vi "build_PWM_task.vi"(0 "counter":string="Dev1/ctr0", 1 "idle state":i32(ring)=10214 items=["High"=10192, "Low"=10214], 2 "initial delay":dbl format="%^.2e", 3 "sample mode":i32(ring)=10178 items=["Finite Samples"=10178, "Continuous Samples"=10123, "Hardware Timed Single Point"=12522], 5 "channel name":string="pwm out", 7 "low time":dbl=0.01 format="%0.2e", 9 "high time":dbl=0.01 format="%0.2e", 11 "error in":errorcluster caption="错误输入", 12 "units":i32(ring)=10364 items=["Seconds"=10364, "From Custom Scale"=10065], 13 "number of samples":i32=100) -> (4 "task out":refnum<k21> caption="任务输出", 15 "error out":errorcluster caption="错误输出")   [LabVIEW 2013]
uses:
  <vilib>/DAQmx/configure/timing.llb/DAQmx Timing (Implicit).vi
  <vilib>/DAQmx/create/channels.llb/DAQmx Create Channel (CO-Pulse Generation-Time).vi
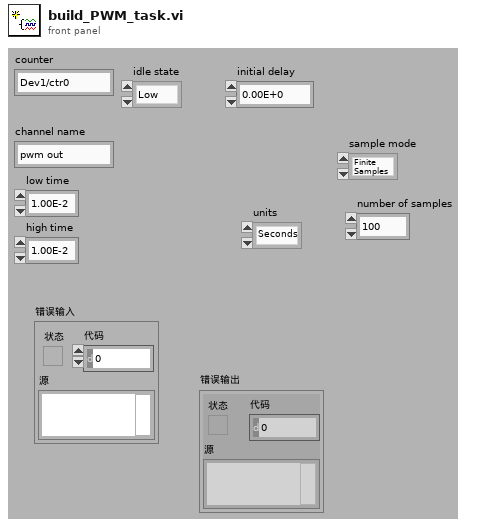
[diagram p1: front panel]
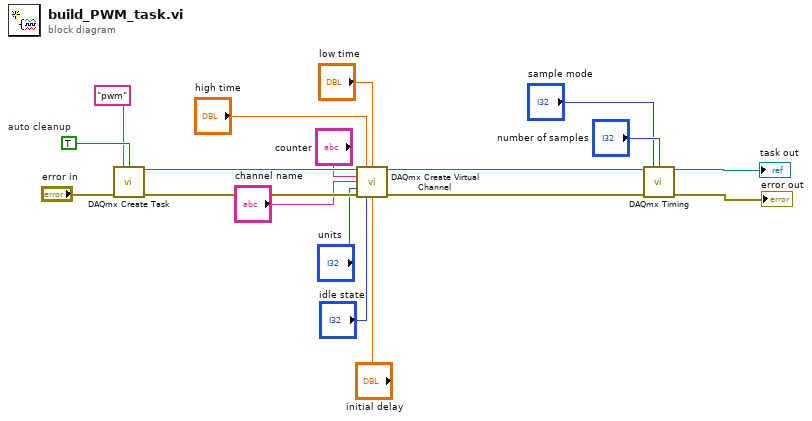
[diagram p0: block diagram]
diagram:
  w16 = TRUE  # auto cleanup
  n1 = call <vilib>:"DAQmx Create Task.vi"("new task name"="pwm", "auto cleanup"=w16, "error in"="error in") -> ("task out"=w15:refnum<k21>, "error out"=w17:errorcluster)  [unwired: 11 in]
  n2 = call-poly <vilib>:"DAQmx Create Virtual Channel.vi"("task in"=w15, "high time"="high time", "low time"="low time", "counter"="counter", "name to assign"="channel name", "units"="units", "error in"=w17, "idle state"="idle state", "initial delay"="initial delay") -> ("task out"=w4:refnum<k21>, "error out"=w13:errorcluster)  [unwired: 5 in]
  n3 = call-poly <vilib>:"DAQmx Timing.vi"("task/channels in"=w4, "sample mode"="sample mode", "samples per channel"="number of samples", "error in"=w13) -> ("task out"=→"task out":refnum<k21>, "error out"=→"error out":errorcluster)  [unwired: 10 in]
